vi "z_n__v1.vi"(7 "n":ext, 8 "ƒÁ[n-1]":ext format="%#.6g", 9 "c[n]":ext format="%#.6g", 10 "b[n]":ext format="%#.6g", 11 "a[n]":ext format="%#.6g") -> (3 "z[n]":ext format="%#.6g")   [LabVIEW 2020]
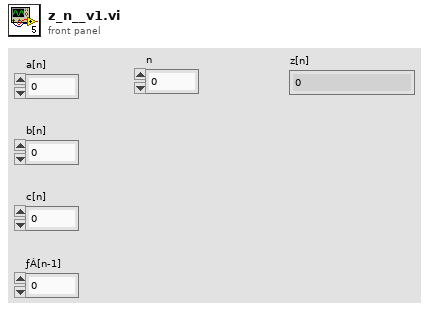
[diagram p1: front panel]
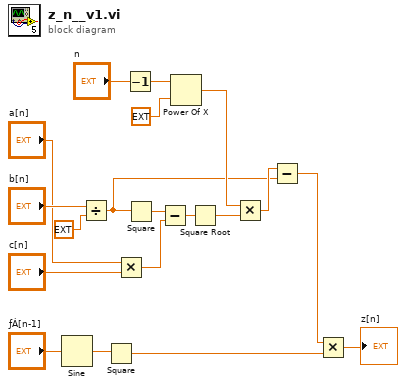
[diagram p0: block diagram]
diagram:
  n1 = Sine(x="ƒÁ[n-1]") -> (sin(x)=w10:ext)
  n2 = Divide(x="b[n]", y=ext 2.0) -> (x/y=w2:ext)
  n3 = Square(x=w10) -> (x^2=w6:ext)
  n4 = Multiply(x="a[n]", y="c[n]") -> (x*y=w14:ext)
  n5 = Decrement(x="n") -> (x-1=w5:ext)
  n6 = Square(x=w2) -> (x^2=w15:ext)
  n7 = Subtract(x=w15, y=w14) -> (x-y=w13:ext)
  n8 = Power Of X(1:ext -1.0, 2:w5) -> (0:w7:ext)
  n9 = Square Root(x=w13) -> (sqrt(x)=w8:ext)
  n10 = Multiply(x=w7, y=w8) -> (x*y=w3:ext)
  n11 = Subtract(x=w3, y=w2) -> (x-y=w1:ext)
  n12 = Multiply(x=w1, y=w6) -> (x*y=→"z[n]":ext)
